vi "BallandBeam(WithLPF).vi"() -> ()   [LabVIEW 2014]
uses:
  <vilib>/myRIO/Instrument Drivers/Onboard IO/AI/vis/Read.vi
  <vilib>/myRIO/Instrument Drivers/Onboard IO/AO/vis/Write.vi
  <vilib>/myRIO/Instrument Drivers/Onboard IO/AI/vis/Smart Open.vi
  <vilib>/Utility/error.llb/Error Cluster From Error Code.vi
  <vilib>/myRIO/Common/Instrument Driver Framework/myRIO v1.0/AI/vis/myRIO v1.0 Read AI.vi
  <vilib>/myRIO/Instrument Drivers/Onboard IO/AO/vis/Smart Open.vi
  <vilib>/myRIO/Common/Instrument Driver Framework/myRIO v1.0/AO/vis/myRIO v1.0 Write AO.vi
panel:
  in  "stop":bool
  out "X voltage":dbl
  out "Theta voltage":dbl
  in  "x amp":dbl=-21.47
  in  "x offset":dbl=96.61
  out "Position":dbl
  in  "t amp":dbl=45.0
  in  "t offset":dbl=-338.2
  out "Theta":dbl
  in  "Sampling rate(Hz)":dbl=50.0
  in  "Kp1":dbl=5.0
  in  "Vout Bound":dbl=4.5
  out "Vout":dbl
  in  "X disire":dbl
  in  "Kd":dbl
  in  "Kp":dbl=0.5
  in  "Theta Bound":dbl=3.0
  out "X Error 2":dbl(graph)=-0.6885397082002527
  out "X Error":dbl
  out "Theta Output":dbl
  in  "Ki":dbl=5.0
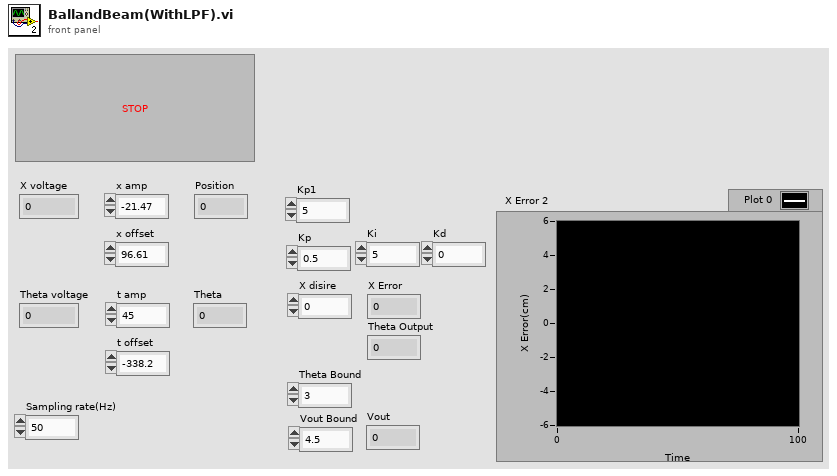
[diagram p1: front panel]
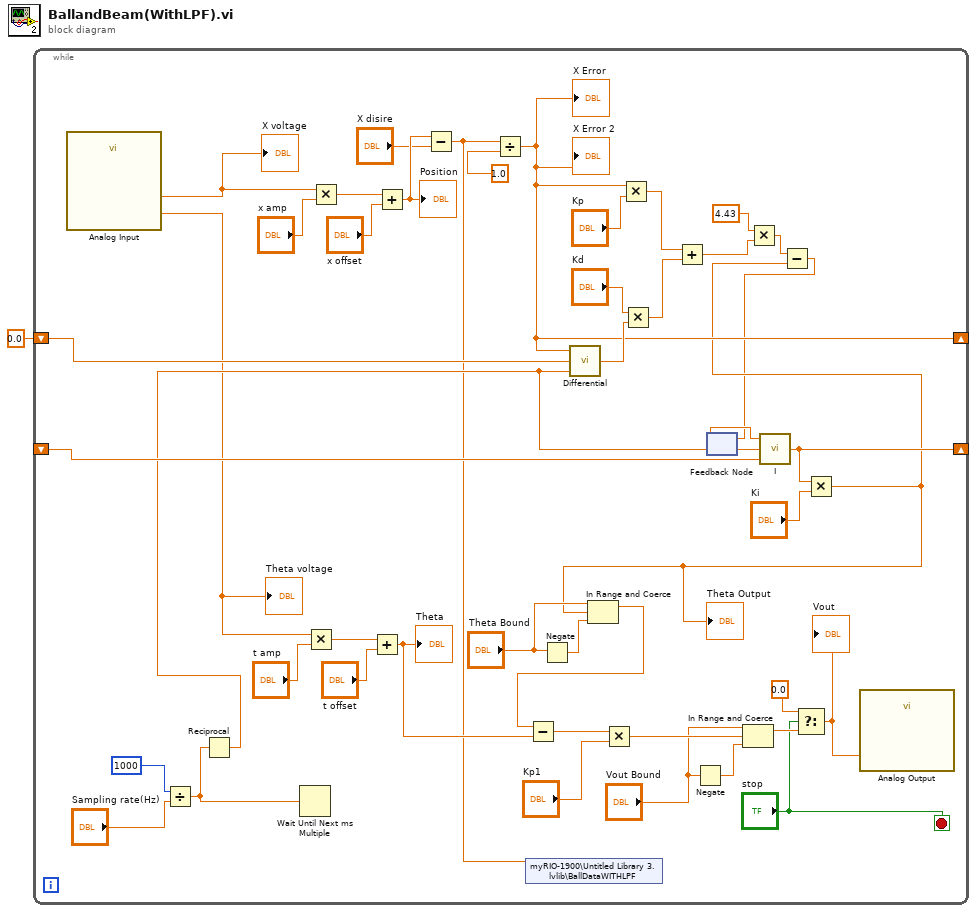
[diagram p0: block diagram]
diagram:
  n1 = while {
    shift-right: [w11] -> _
    shift-left: 0.0 -> [w23]
    shift-right: [w15] -> _
    shift-left: _ -> [w16]
    stop <- "stop" stop-if-true
    n2 = call "Analog Input"() -> ("C/AI0"=w4:dbl, "C/AI1"=w3:dbl)  [unwired: 25 in, 1 out]
    "X voltage" <- w4
    "Theta voltage" <- w3
    n3 = Divide(x=1000, y="Sampling rate(Hz)") -> (x/y=w29:dbl)
    n4 = Reciprocal(x=w29) -> (1/x=w13:dbl)
    n5 = Wait Until Next ms Multiple(millisecond multiple=w29) -> ()  [unwired: 1 out]
    n6 = Multiply(x=w3, y="t amp") -> (x*y=w43:dbl)
    n7 = Multiply(x=w4, y="x amp") -> (x*y=w46:dbl)
    n8 = Add(x=w43, y="t offset") -> (x+y=w31:dbl)
    "Theta" <- w31
    n9 = Add(x=w46, y="x offset") -> (x+y=w19:dbl)
    "Position" <- w19
    n10 = Subtract(x=w19, y="X disire") -> (x-y=w10:dbl)
    n11 = Divide(x=w10, y=1.0) -> (x/y=w11:dbl)
    "X Error 2" <- w11
    "X Error" <- w11
    n12 = shared-variable "myRIO-1900\\Untitled Library 3.lvlib\\BallDataWITHLPF"(w10) -> ()  [unwired: 1 in, 1 out]
    n13 = Negate(x="Theta Bound") -> (-x=w21:dbl)
    n14 = call "Differential.vi"("Ts"=w13, "X[k-1]"=w23, "X[k]"=w11) -> ("dX"=w28:dbl)
    n15 = Multiply(x=w11, y="Kp") -> (x*y=w25:dbl)
    n16 = Multiply(x="Kd", y=w28) -> (x*y=w24:dbl)
    n17 = Add(x=w25, y=w24) -> (x+y=w6:dbl)
    n18 = Negate(x="Vout Bound") -> (-x=w36:dbl)
    n19 = feedback #1() -> (w14:dbl)  [unwired: 1 in]
    n20 = Multiply(x=4.43 ("y"), y=w6) -> (x*y=w5:dbl)
    n21 = call "I.vi"("sum[k-1]"=w16, "Ts"=w13, "error"=w14) -> ("sum"=w15:dbl)
    n22 = Multiply(x=w15, y="Ki") -> (x*y=w9:dbl)
    "Theta Output" <- w9
    n23 = In Range and Coerce(upper limit="Theta Bound", x=w9, lower limit=w21) -> (coerced(x)=w20:dbl)  [unwired: 1 out]
    n24 = Subtract(x=w20, y=w31) -> (x-y=w30:dbl)
    n25 = Multiply(x=w30, y="Kp1") -> (x*y=w35:dbl)
    n26 = In Range and Coerce(upper limit="Vout Bound", x=w35, lower limit=w36) -> (coerced(x)=w34:dbl)  [unwired: 1 out]
    n27 = Subtract(x=w5, y=w9) -> (x-y=w8:dbl)
    n28 = feedback-in #1(w8) -> ()
    n29 = Select(t=0.0, s="stop", f=w34) -> (s? t:f=w2:dbl)
    "Vout" <- w2
    n30 = call "Analog Output"("C/AO0"=w2) -> ()  [unwired: 26 in, 1 out]
  }
